vi "Discrete PID.vi"(4 "Gains Motor 1":dbl[](array[numeric]), 6 "Gains Motor 0":dbl[](array[numeric]), 11 "Error Array":dbl[](array[numeric])) -> (3 "Voltage":dbl[](array[numeric]))   [LabVIEW 2019]
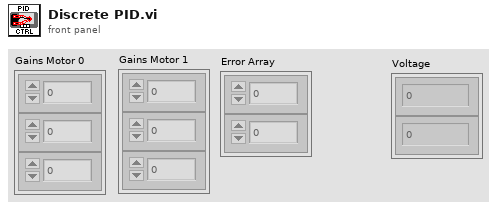
[diagram p1: front panel]
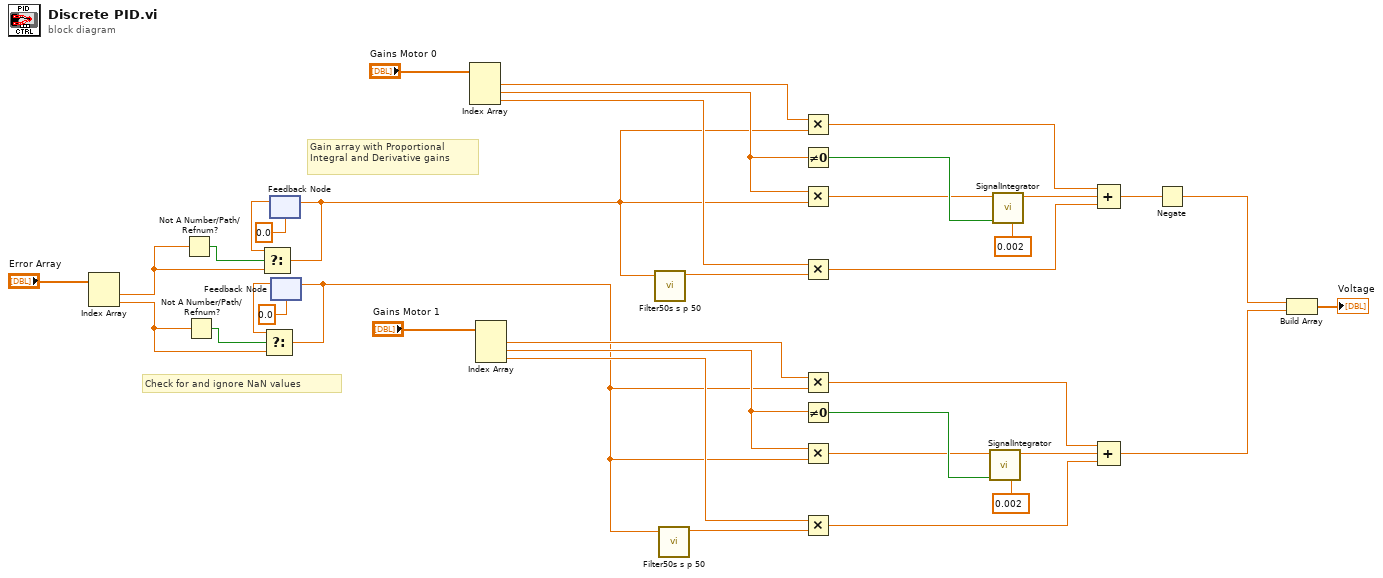
[diagram p0: block diagram]
diagram:
  # "Check for and ignore NaN values"
  # "Gain array with Proportional\nIntegral and Derivative gains"
  n1 = Index Array ("Index Array 4")(array="Error Array") -> (element #1=w5:dbl, element #2=w4:dbl)  [unwired: 2 in]
  n2 = Not A Number/Path/Refnum?(number/path/refnum=w5) -> (NaN/Path/Refnum?=w10:bool)
  n3 = Not A Number/Path/Refnum? ("Not A Number/Path/Refnum? 2")(number/path/refnum=w4) -> (NaN/Path/Refnum?=w7:bool)
  n4 = feedback #1(0.0 ("Input")) -> (w11:dbl)
  n5 = Select(t=w11, s=w10, f=w5) -> (s? t:f=w3:dbl)
  n6 = feedback-in #1 ("2")(w3) -> ()
  n7 = feedback #2 ("Feedback Node 2")(0.0 ("Input 2")) -> (w8:dbl)
  n8 = Select ("Select 2")(t=w8, s=w7, f=w4) -> (s? t:f=w2:dbl)
  n9 = feedback-in #2 ("3")(w2) -> ()
  n10 = Index Array ("Index Array 2")(array="Gains Motor 0") -> (element #1=w30:dbl, element #2=w28:dbl, element #3=w27:dbl)  [unwired: 3 in]
  n11 = Index Array ("Index Array 3")(array="Gains Motor 1") -> (element #1=w25:dbl, element #2=w23:dbl, element #3=w22:dbl)  [unwired: 3 in]
  n12 = call "Filter50s s p 50.vi"("u"=w3) -> ("y"=w26:dbl)  [unwired: 10 in]
  n13 = call "Filter50s s p 50.vi"("u"=w2) -> ("y"=w21:dbl)  [unwired: 10 in]
  n14 = Multiply(x=w30, y=w3) -> (x*y=w19:dbl)
  n15 = Not Equal To 0?(x=w28) -> (x != 0?=w34:bool)
  n16 = Multiply ("Multiply 2")(x=w28, y=w3) -> (x*y=w29:dbl)
  n17 = Multiply ("Multiply 3")(x=w27, y=w26) -> (x*y=w17:dbl)
  n18 = Multiply ("Multiply 4")(x=w25, y=w2) -> (x*y=w15:dbl)
  n19 = Not Equal To 0? ("Not Equal To 0? 2")(x=w23) -> (x != 0?=w31:bool)
  n20 = Multiply ("Multiply 5")(x=w23, y=w2) -> (x*y=w24:dbl)
  n21 = Multiply ("Multiply 6")(x=w22, y=w21) -> (x*y=w13:dbl)
  n22 = call "SignalIntegrator.vi"("Ts"=0.002 ("Ts 2"), "Reset"=w31, "x"=w24) -> ("y"=w14:dbl)  [unwired: 8 in]
  n23 = call "SignalIntegrator.vi"("Ts"=0.002, "Reset"=w34, "x"=w29) -> ("y"=w18:dbl)  [unwired: 8 in]
  n24 = Compound Arithmetic op=ADD(w19, w18, w17) -> (w16:dbl)
  n25 = Compound Arithmetic op=ADD ("Compound Arithmetic 2")(w15, w14, w13) -> (w12:dbl)
  n26 = Negate(x=w16) -> (-x=w20:dbl)
  n27 = Build Array ("Build Array 4")(w20, w12) -> (→"Voltage":dbl[])
